vi "Add Found xVDT to Array.vi"(7 "Index Found":i32, 8 "Controls In":T1[](array[typedef]), 9 "ScaleFactor 1 Name":string, 10 "xVDT Number":string, 11 "xVDTs In":T2[](array[typedef])) -> (2 "Controls Out":T1[](array[typedef]), 3 "xVDTs Out":T2[](array[typedef]), 5 "Next Index":i32)   [LabVIEW 2010, in "Sensor Simulation Custom Device.lvlib"]
uses:
  Sensor Simulation Custom Device.lvlib
  <userlib>/_FPGA Interface Advanced Tools/FPGA Bitfile Utility/TypeDefs/Scalar Register.ctl
  TypeDefs/xVDT.ctl
  <userlib>/_FPGA Interface Advanced Tools/FPGA Bitfile Utility/FPGA Bitfile Utility.lvlib
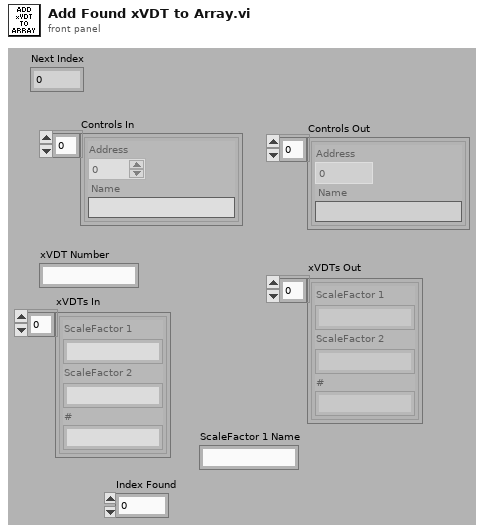
[diagram p1: front panel]
types:
  T1 = typedef "FPGA Bitfile Utility.lvlib/Scalar Register.ctl" = cluster{"Address":u32, "Name":string}
  T2 = typedef "Sensor Simulation Custom Device.lvlib/xVDT.ctl" = cluster{"ScaleFactor 1":string, "ScaleFactor 2":string, "#":string}
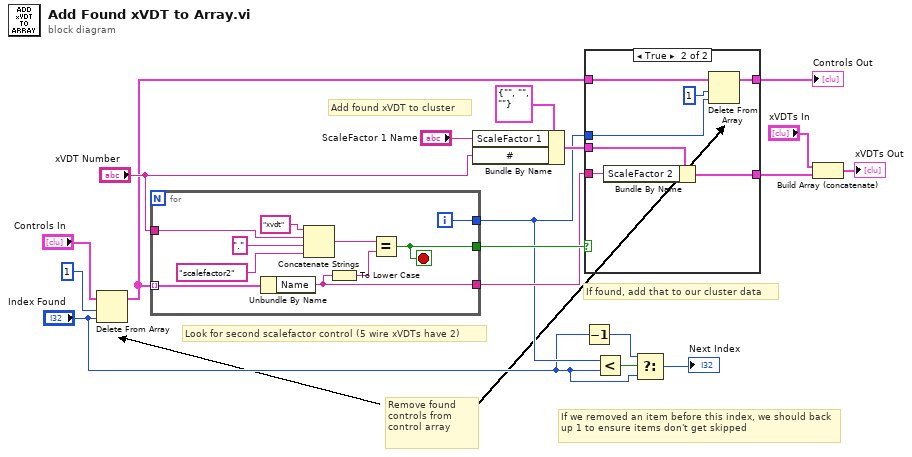
[diagram p0: block diagram]
diagram:
  # "If we removed an item before this index, we should back up 1 to ensure items don't get skipped"
  # "Remove found controls from control array"
  # "If found, add that to our cluster data"
  # "Look for second scalefactor control (5 wire xVDTs have 2)"
  # "Add found xVDT to cluster"
  n1 = Delete From Array(array="Controls In", length=1, index="Index Found") -> (array with subset deleted=w7:T1[])  [unwired: 1 out]
  n2 = for {
    tunnel: [w22] -> w12
    tunnel: [w24] -> w10
    tunnel: [w23] -> w3
    tunnel: w7 -> [w19] mode=indexing
    tunnel: "xVDT Number" -> [w21]
    i -> [w23]
    stop <- w22 stop-if-true
    n3 = Unbundle By Name(w19) -> ("Name"=w24:string)
    n4 = Concatenate Strings("xvdt" ("regular expression"), w21, "." ("string"), "scalefactor2" ("regular expression")) -> (w25:string)
    n5 = To Lower Case(string=w24) -> (all lower case string=w28:string)
    n6 = Equal?(x=w25, y=w28) -> (x = y?=w22:bool)
  }
  n7 = Bundle By Name(cluster=T2 {"ScaleFactor 1"="", "ScaleFactor 2"="", "#"=""}, "ScaleFactor 1"="ScaleFactor 1 Name", "#"="xVDT Number") -> (w11:T2)
  n8 = Decrement(x="Index Found") -> (x-1=w2:i32)
  n9 = case shown="True" w12 {
    tunnel: w11 -> [w30 w37]
    tunnel: w10 -> [_ w36]
    tunnel: [w30 w35] -> w9
    tunnel: w7 -> [w29 w33]
    tunnel: w3 -> [_ w32]
    tunnel: [w29 w31] -> w6
    frame False {
    }
    frame True {
      n10 = Bundle By Name(cluster=w37, "ScaleFactor 2"=w36) -> (w35:T2)
      n11 = Delete From Array(array=w33, length=1, index=w32) -> (array with subset deleted=w31:T1[])  [unwired: 1 out]
    }
  }
  "Controls Out" <- w6
  n12 = Less?(x=w3, y="Index Found") -> (x < y?=w5:bool)
  n13 = Select(t=w2, s=w5, f="Index Found") -> (s? t:f=→"Next Index":i32)
  n14 = Build Array (concatenate)("xVDTs In", w9) -> (→"xVDTs Out":T2[])
